vi "calcula brewster.vi"(6 "Ángulo Final":dbl, 9 "Ángulo Inicial":dbl, 10 "EJE Y":dbl[](array[numeric]), 11 "EJE X":dbl[](array[numeric])) -> (1 "Ángulo de Brewster":dbl, 2 "Curva FILTRADA":cluster{dbl[], dbl[]}(graph), 3 "Curva de reflectancia":cluster{dbl[], dbl[]}(graph), 4 "Índice de Refracción":dbl, 5 "Numeric Control":dbl)   [LabVIEW 2025]
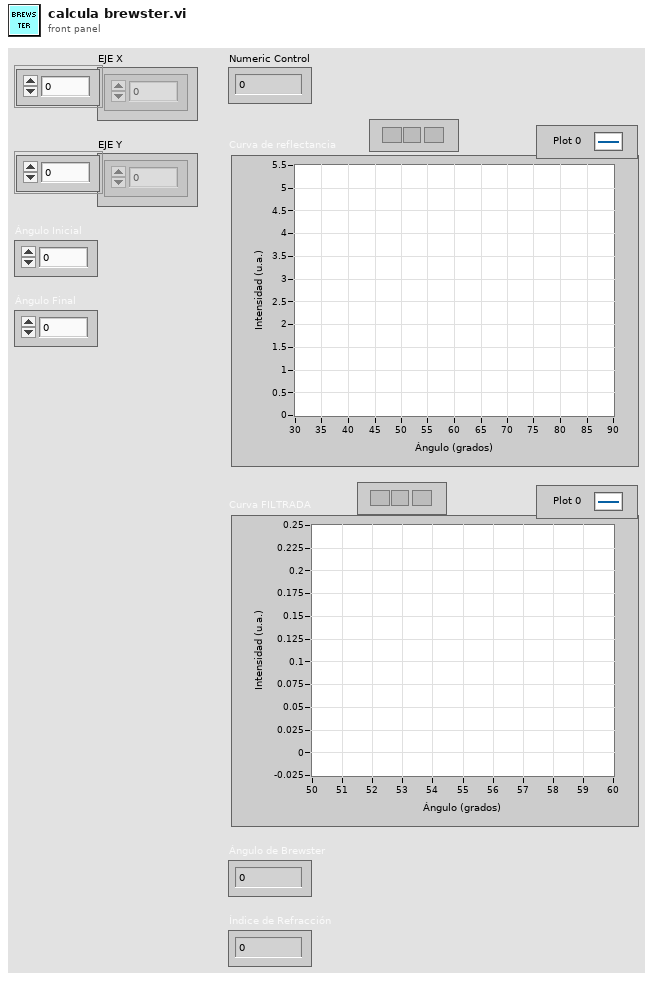
[diagram p1: front panel]
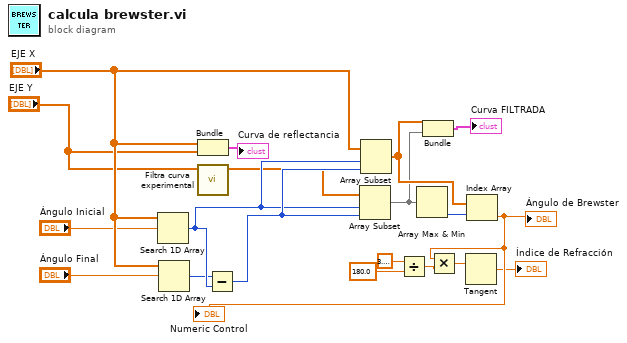
[diagram p0: block diagram]
diagram:
  n1 = Search 1D Array(1D array="EJE X", element="Ángulo Inicial") -> (index of element=w8:i32)  [unwired: 1 in]
  n2 = Search 1D Array(1D array="EJE X", element="Ángulo Final") -> (index of element=w7:i32)  [unwired: 1 in]
  n3 = Bundle("EJE X"="EJE X", "EJE Y"="EJE Y") -> (→"Curva de reflectancia":cluster{"EJE X":dbl[], "EJE Y":dbl[]})  [unwired: 1 in]
  n4 = call "Filtra curva experimental.vi"("Y"="EJE Y") -> ("Y Filtrada"=w3:dbl[])  [unwired: 8 in, 2 out]
  n5 = Subtract(x=w7, y=w8) -> (x-y=w9:i32)
  n6 = Array Subset(array=w3, index=w8, length=w9) -> (w1:dbl[])
  n7 = Array Subset(array="EJE X", index=w8, length=w9) -> (w2:dbl[])
  n8 = Divide(x=3.141592653589793, y=180.0) -> (x/y=w16:dbl)
  n9 = Array Max & Min(array=w1) -> (min index (indices)=w12:i32)  [unwired: 3 out]
  n10 = Bundle(w2, w1) -> (→"Curva FILTRADA":cluster{dbl[], dbl[]})  [unwired: 1 in]
  n11 = Index Array(array=w2, index=w12) -> (element=w19:dbl)
  "Ángulo de Brewster" <- w19
  "Numeric Control" <- w19
  n12 = Multiply(x=w19, y=w16) -> (x*y=w17:dbl)
  n13 = Tangent(1:w17) -> (0:→"Índice de Refracción":dbl)
